vi "Find Dependency Chain.vi"() -> ()   [LabVIEW 2019, in "HawkeyeToolsMenu.lvlib"]
doc: "GUI to compare LabVIEW code between currently checked out branch with any other branch or any of its commits.\n\n(c) 2024 Soliton Technologies. All rights reserved."
uses:
  HawkeyeToolsMenu.lvlib
  cd7db559-2e0e-4359-8ea8-99399200914e.vi
  74b97984-16df-4a5a-bd9d-c6fa6725c391.vi
  vi.lib/Hawkeye/Hawkeye.lvlib
panel:
  in  "Tab Control":T1(tab)=enum."Main UI"
  out "Dependency Chain":string
  in  "Selected Dependencies":string(combo)="origin/main" caption="Dependencies"
  in  "Stop":bool
  in  "lvlib / class Path":path
  # "1. Checkout the branch of interest in your system using any method - Git command line, Desktop Git GUI Clients etc.,\n\n2. Specify the local Repository Path.\n\n3. Verify the current branch, its status and select a branch or commit based on the Compare Mode and click on Compare to display the file changes.\n\n4. Double click on a file to initiate LabVIEW code comparison.\n\n5. Once done with required comparisons, exit the tool by closing the window. The tool cleans up the temporary files added during comparison.\n\n\nNote:\n1. This tool uses LabVIEW's VI Comparison Tool which requires LabVIEW Professional Development System.\n2. It is recommended to not use other Git Clients actively when comparing files using this tool to avoid Git command related errors.\n3. It is recommended to commit all changes (working copy) before using this tool for comparison."
  # "This tool uses git diff command to identify the changes. Hence it is recommended to commit all the changes (working copy) to have them considered for comparison. For code comparison, this tool uses LabVIEW's built in VI Comparison Tool.\n\nExample: Identify changes in current branch when comparing with other branch\n\n---A---B---C---D    <== other branch\n               \\\n                 E---F      <== current branch\n\n1. We will need to identify only the file changes introduced by current branch. E and F commits are those changes in the above example (commits after the common ancestor B).\n2. For the identified file changes compare with the other branch (D) to see how it differs. These differences will be our current branch changelist.\n\nWhy only current branch changes?\nIt is most useful to see how the current branch will modify the files when it is getting merged. Best use case for displaying only current branch changelist will be for Pull Request reviews."
  # "1. VI / lvlib / class Path (Config Path)\n\n    What it is: The starting point of your dependency analysis.\n\n    How to use: Browse to or enter the absolute file path of the LabVIEW file you want to inspect.\n\n    Supported File Types: * Virtual Instruments (.vi) / LabVIEW Project Libraries (.lvlib) / LabVIEW Classes (.lvclass)\n\n2. Dependencies in Linked Project (Dropdown Menu)\n\n    What it is: A dynamically populated dropdown list showing all the valid LabVIEW files found within the scope of your linked project.\n\n    How to use: After configuring your source path, select any file from this dropdown to check if a relationship exists between it and your Config Path.\n\n3. Dependency Chain (Output Display)\n\n    What it is: The visual results area that shows the exact \"calling route\" from your Config Path to the selected dropdown dependency."
  # "Find Dependency Chain\n\nThe LabVIEW Dependency Analyzer is a specialized utility designed to map, trace, and visualize relationships between components within LabVIEW Projects, Libraries (.lvlib), and Classes (.lvclass).\n\nBy performing deep, recursive analysis on your codebase, it helps developers understand structural coupling, identify hidden linkages, and trace execution paths from a chosen source file down to its deepest sub-components.\n\nKey Features\nDeep Tracing: Automatically traverses multi-level call chains, mapping both direct and indirect dependencies."
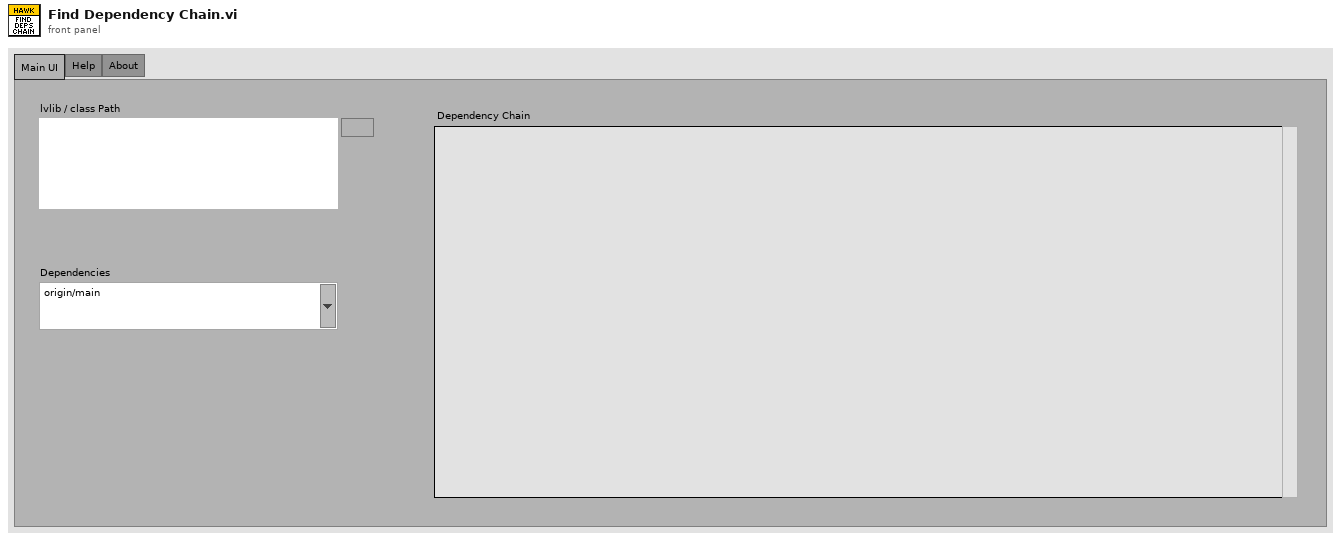
[diagram p1: front panel]
types:
  T1 = enum32{"Getting Started", "How it Works?", "Main UI", "Help", "About"}
  T2 = cluster{"lvlib / class Path":path, "Dependency Start":string, "Dependency End":string, "Repo Path":path, "All Dependency Chain":string, "Dependency Chain []":string[]}
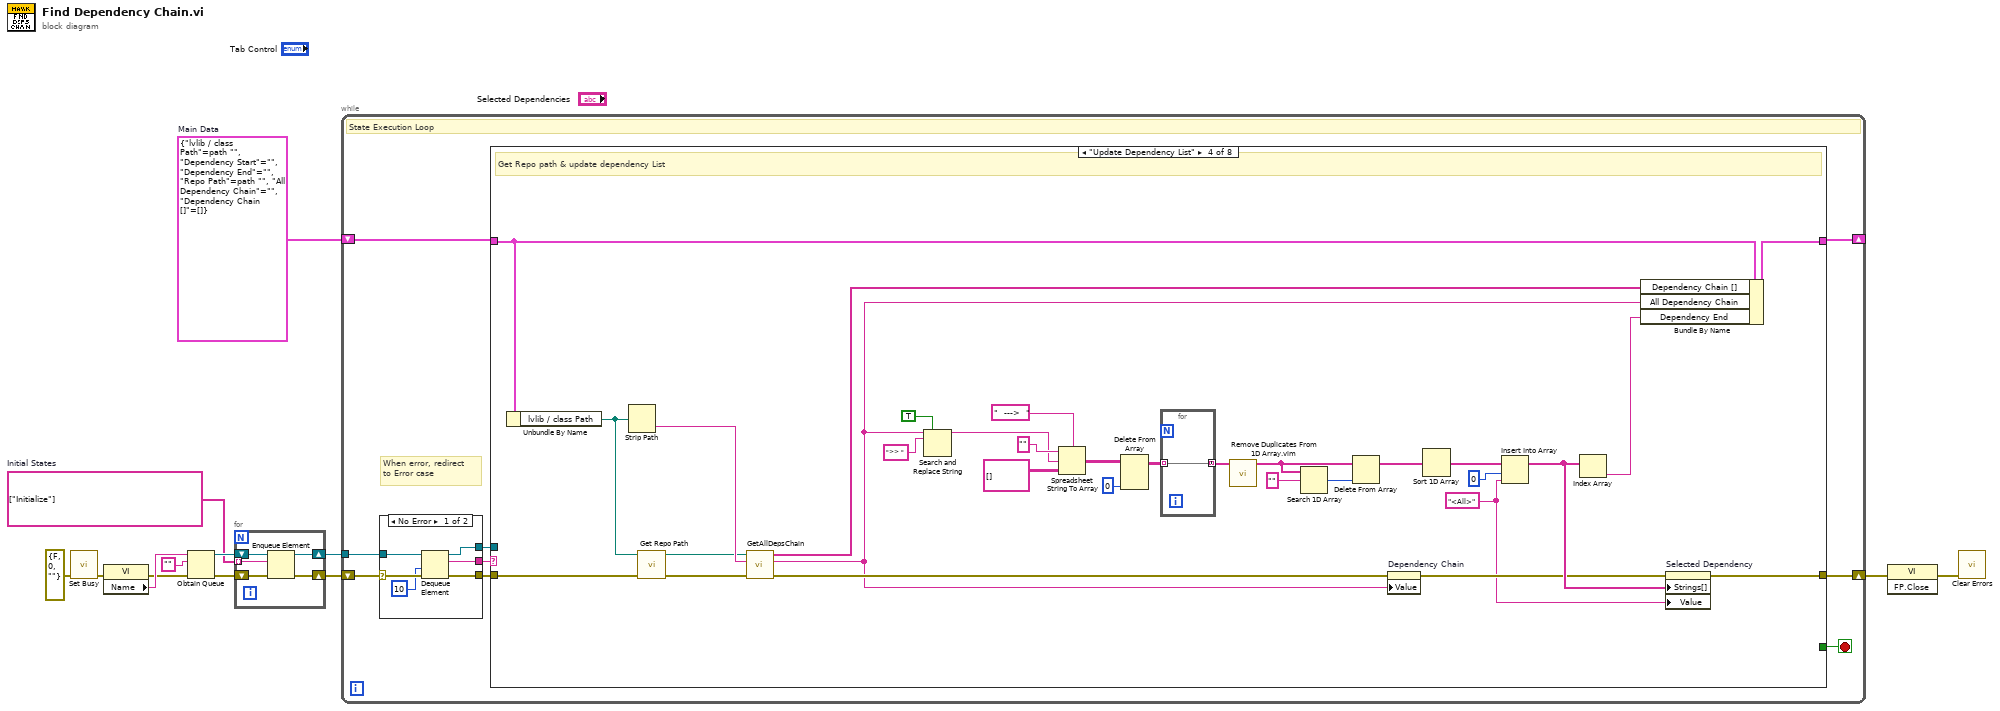
[diagram p0: block diagram]
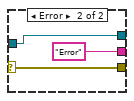
[diagram p2: hidden frame]
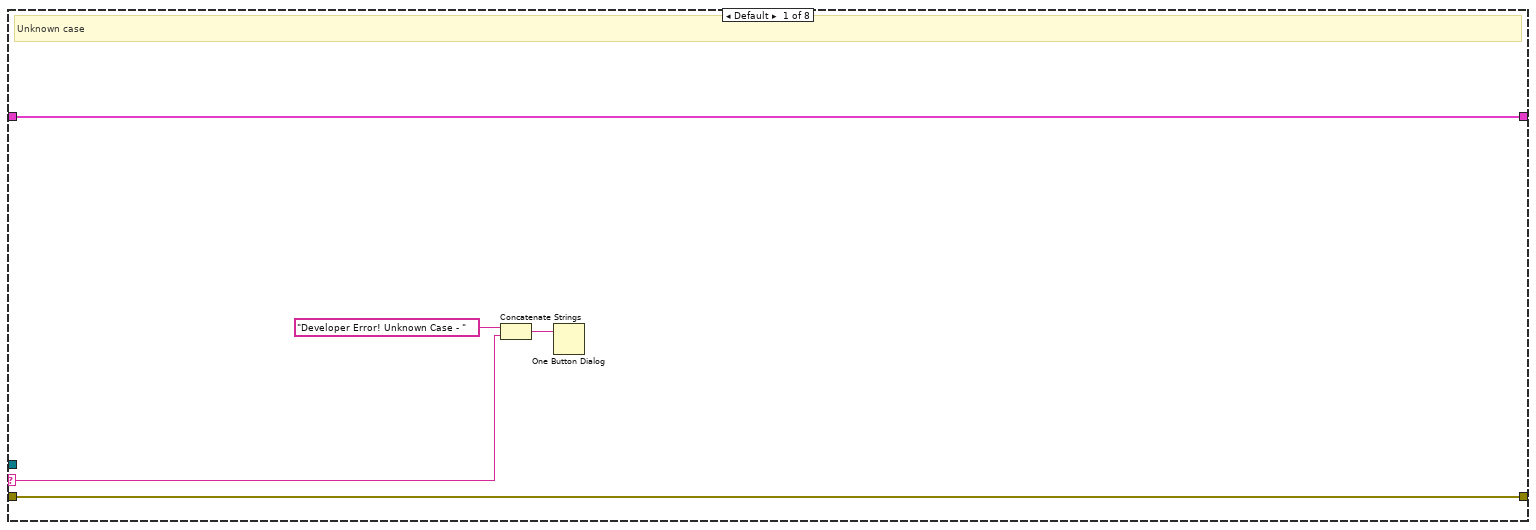
[diagram p3: hidden frame]
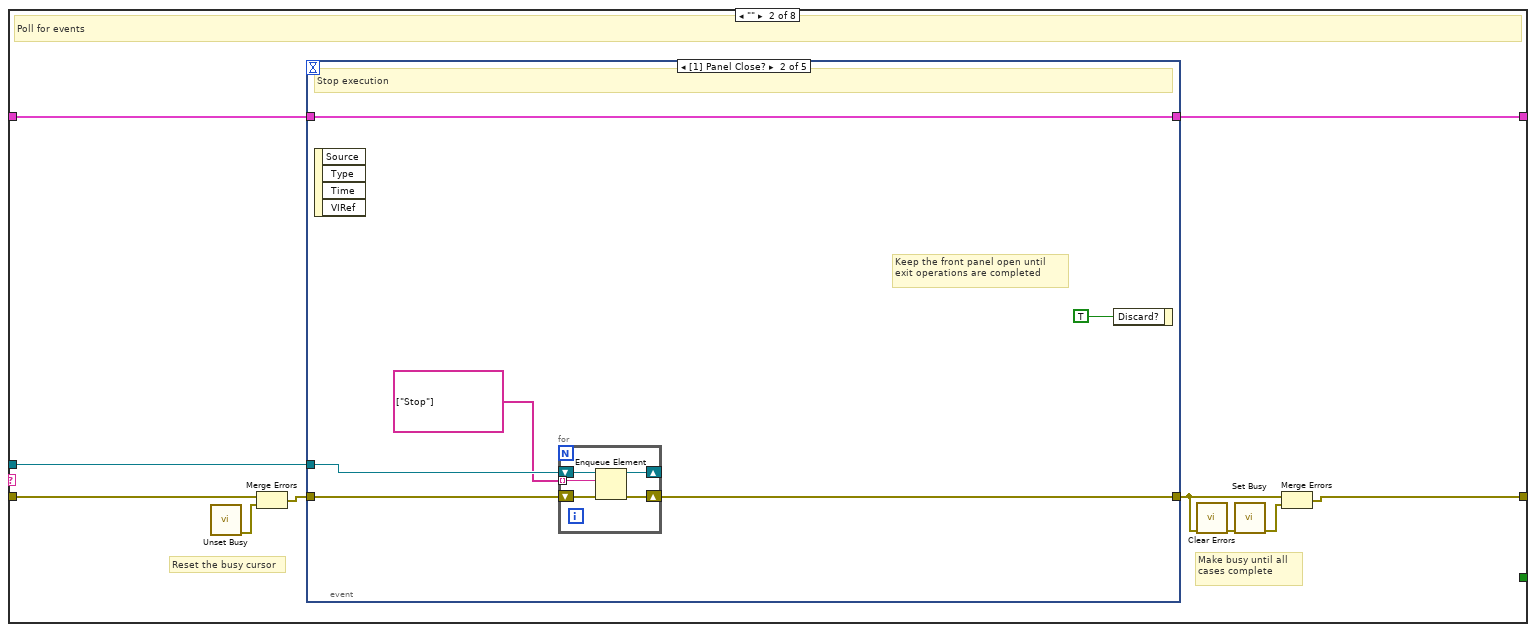
[diagram p4: hidden frame]
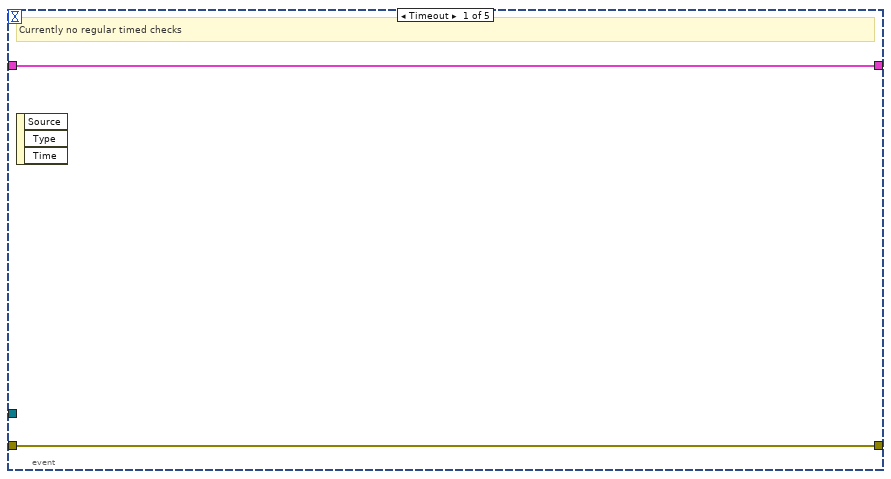
[diagram p5: hidden frame]
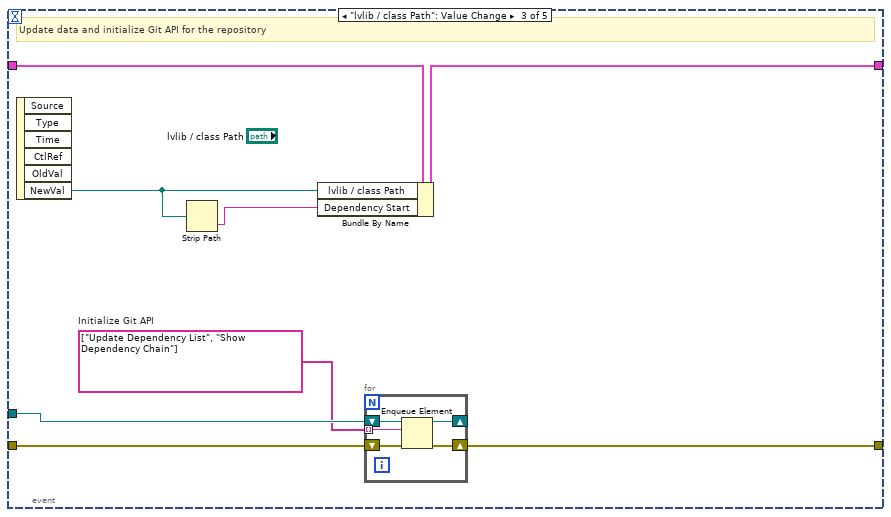
[diagram p6: hidden frame]
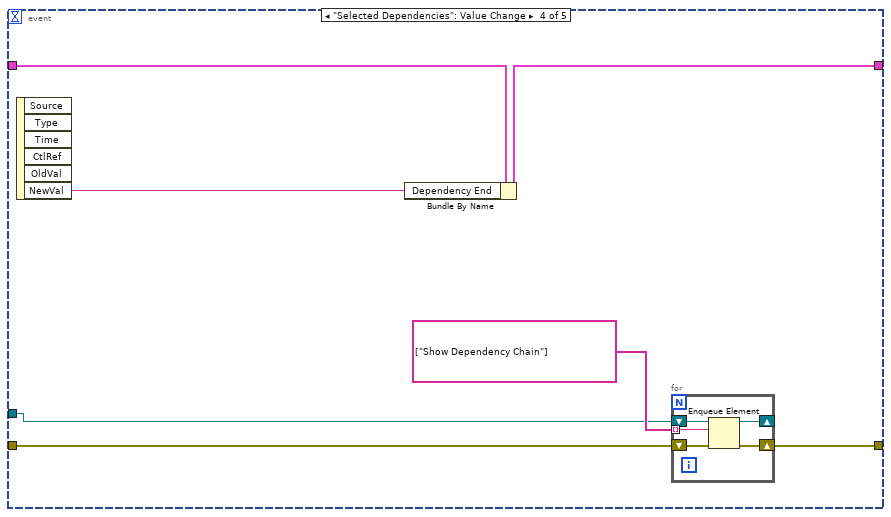
[diagram p7: hidden frame]
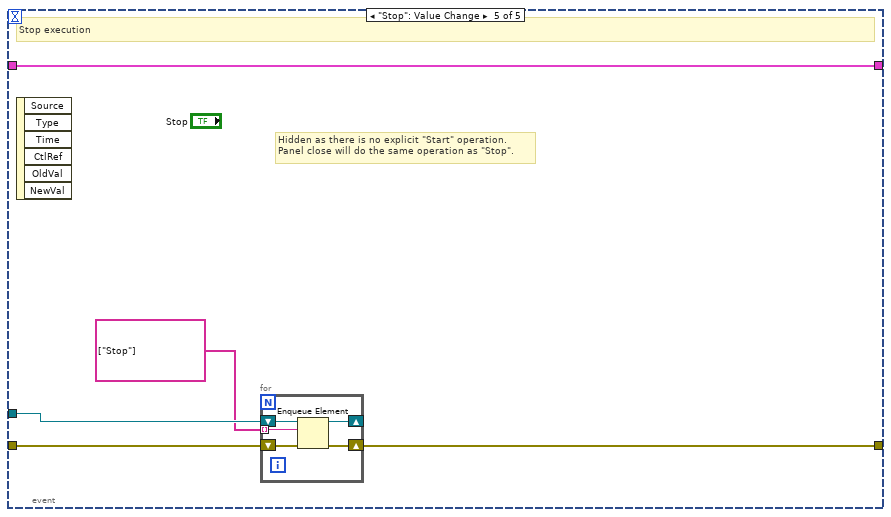
[diagram p8: hidden frame]
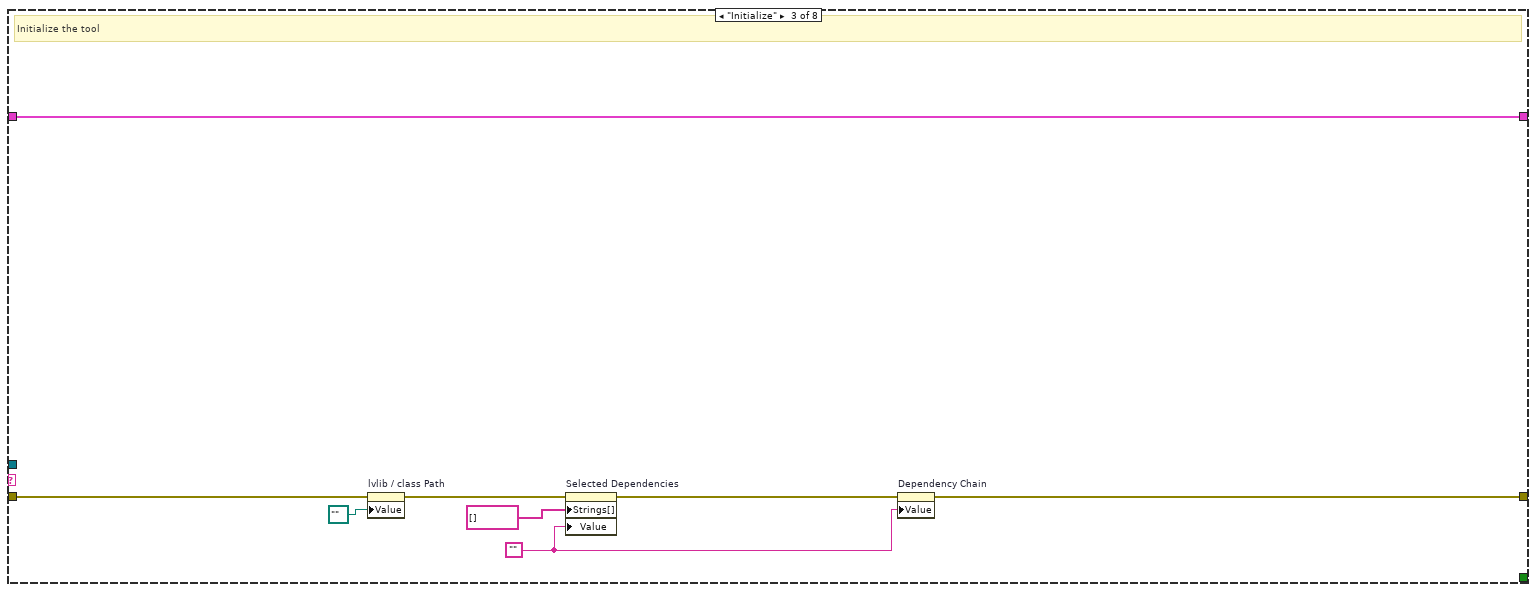
[diagram p9: hidden frame]
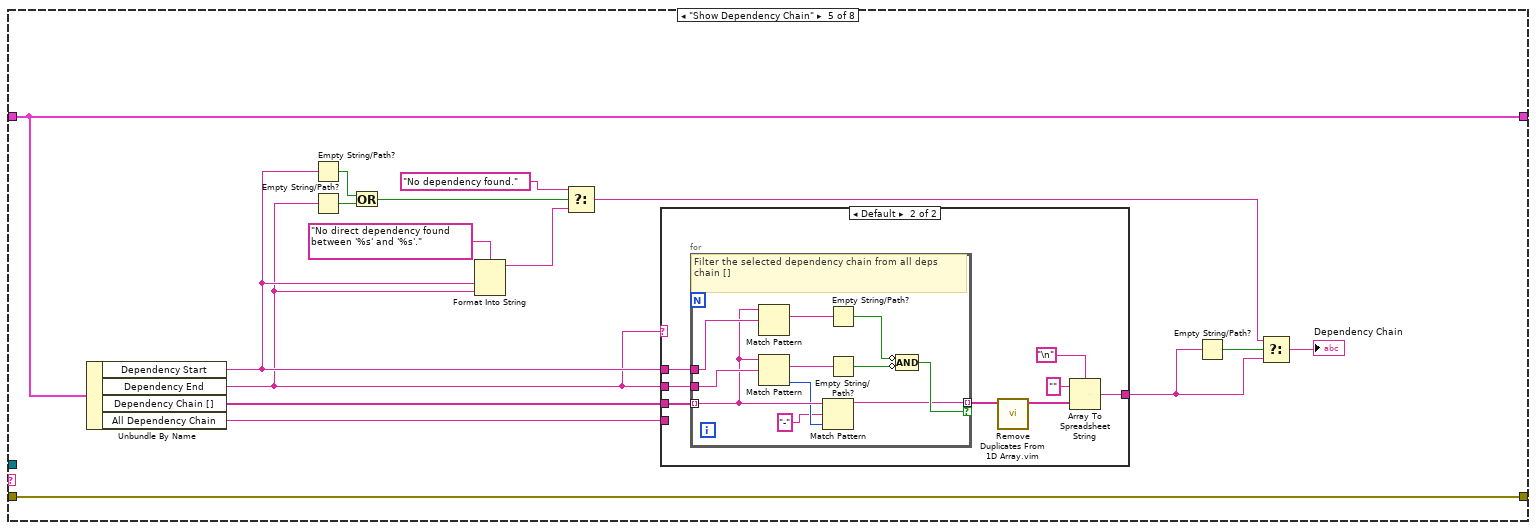
[diagram p10: hidden frame]
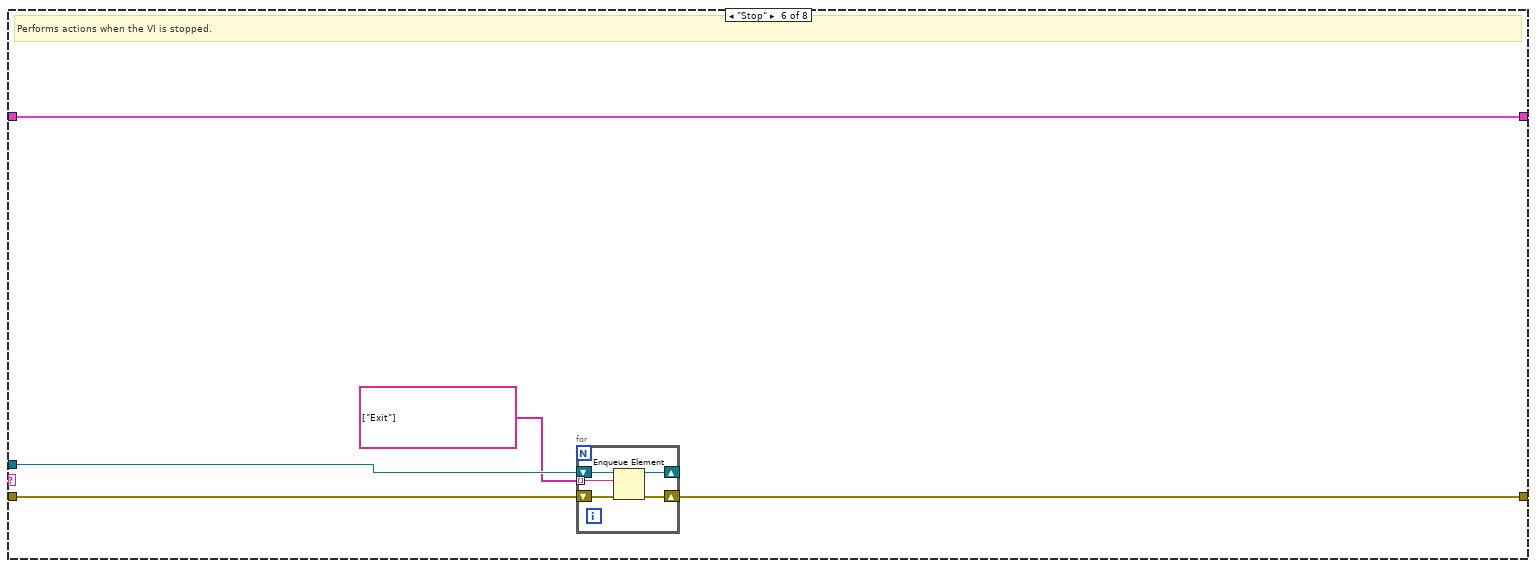
[diagram p12: hidden frame]
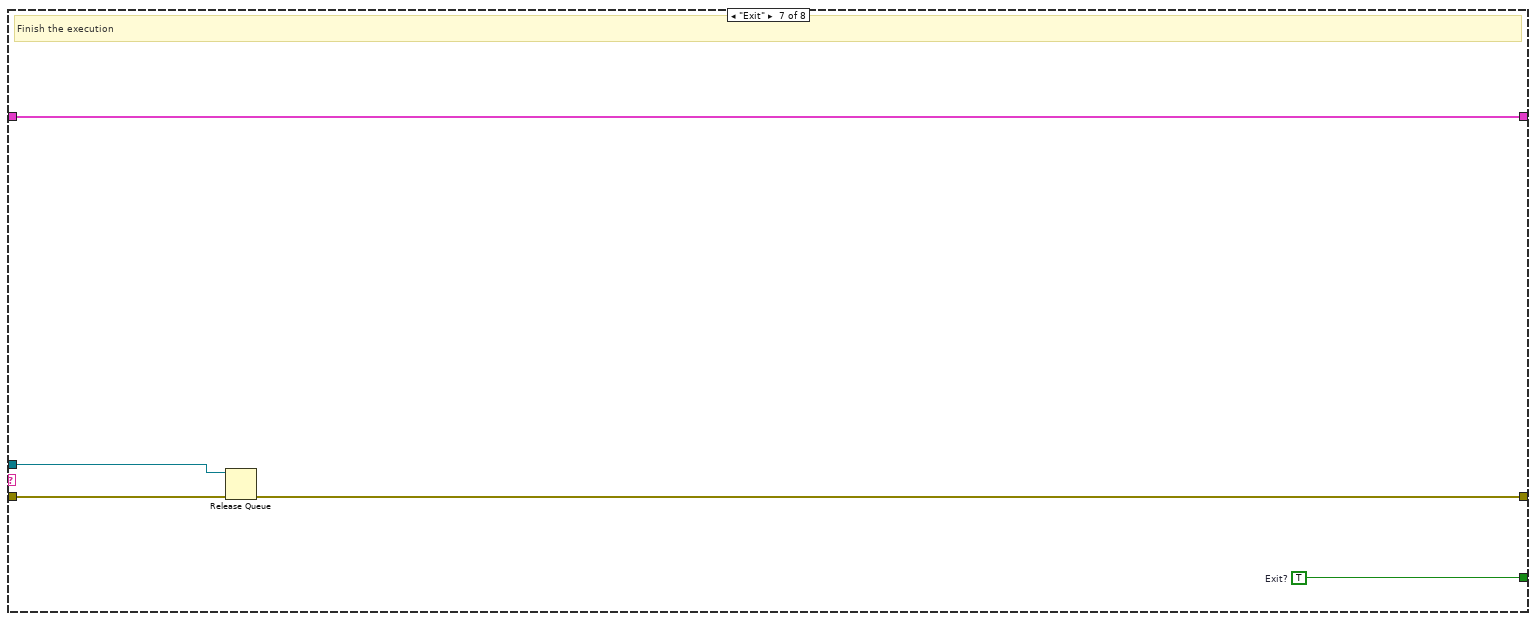
[diagram p13: hidden frame]
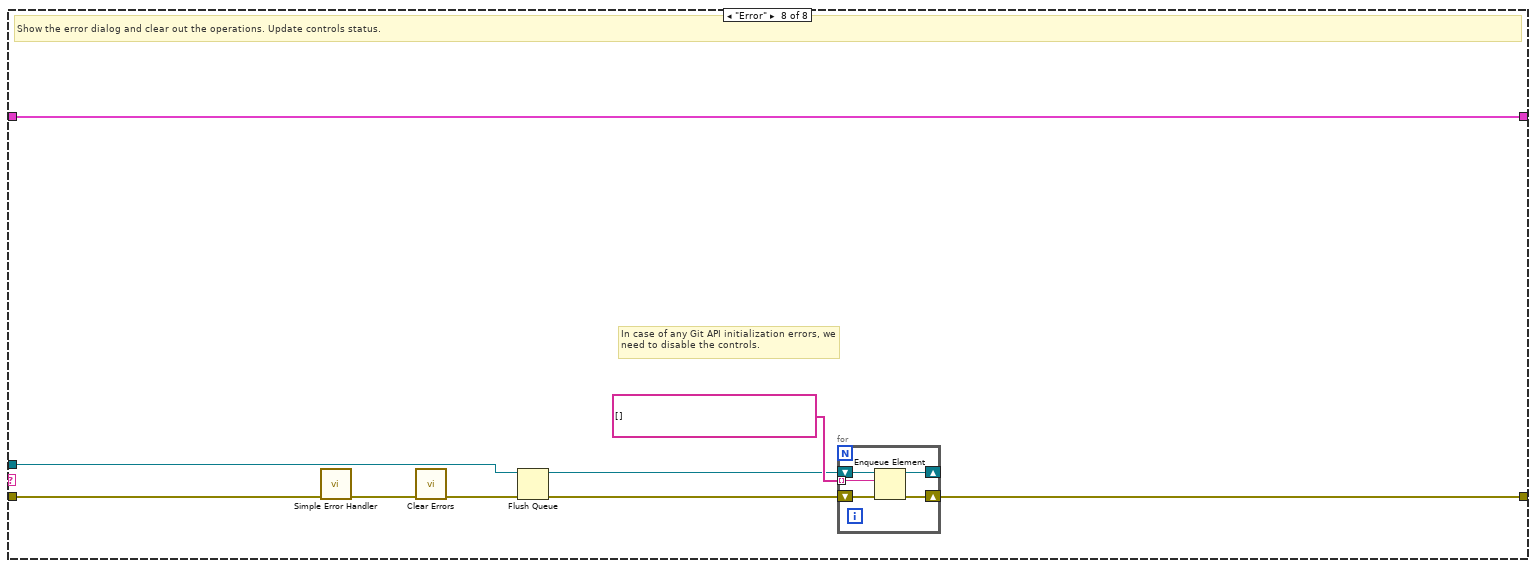
[diagram p14: hidden frame]
diagram:
  w1 = string[] ["Initialize"]  # Initial States
  w10 = T2 {"lvlib / class Path"=path "", "Dependency Start"="", "Dependency End"="", "Repo Path"=path "", "All Dependency Chain"="", "Dependency Chain []"=[]}  # Main Data
  n1 = call <vilib>:"Set Busy.vi"("error in (no error)"=errorcluster {"status"=FALSE, "code"=0, "source"=""}) -> ("error out"=w4:errorcluster)  [unwired: 9 in, 1 out]
  n2 = property class="VI"(error in=w4) -> (error out=w12:errorcluster, "Name"=w13:string)  [unwired: 1 in, 1 out]
  n3 = Obtain Queue(name (unnamed)=w13, element data type="", error in (no error)=w12) -> (queue out=w9:refnum<queue>, error out=w6:errorcluster)  [unwired: 2 in, 1 out]
  n4 = for {
    tunnel: w1 -> [w15] mode=indexing
    shift-right: [w17] -> w8
    shift-left: w6 -> [w18]
    shift-right: [w14] -> w7
    shift-left: w9 -> [w16]
    n5 = Enqueue Element(queue=w16, element=w15, error in (no error)=w18) -> (queue out=w14:refnum<queue>, error out=w17:errorcluster)  [unwired: 1 in, 1 out]
  }
  n6 = while {
    shift-right: [w19] -> w3
    shift-left: w8 -> [w21]
    tunnel: w7 -> [w22]
    shift-right: [w24] -> _
    shift-left: w10 -> [w23]
    stop <- w25 stop-if-true
    # "When error, redirect to Error case"
    # "State Execution Loop"
    n7 = case shown="No Error" w21 {
      selector: w21 -> [w30 w34]
      tunnel: [w33 "Error" ("element")] -> w27
      tunnel: [w32 w36] -> w26
      tunnel: w22 -> [w31 w36]
      tunnel: [w28 w34] -> w20
      frame No Error {
        n8 = Dequeue Element(queue=w31, timeout in ms (-1)=10, error in (no error)=w30) -> (queue out=w32:refnum<queue>, element=w33:string, error out=w28:errorcluster)  [unwired: 1 out]
      }
      frame Error {
      }
    }
    n9 = case shown="\"Update Dependency List\"" w27 {
      selector: w27 -> [w40 _ _ _ _ _ _ _]
      tunnel: w20 -> [w38 w45 w106 w121 w154 w180 w190 w198]
      tunnel: w26 -> [_ w51 _ _ _ w178 w187 w195]
      tunnel: [w38 w47 w100 w137 w154 w179 w186 w191] -> w19
      tunnel: [_ _ _ _ _ _ w188 _] -> w25
      tunnel: [w37 w49 w107 w136 w155 w177 w189 w199] -> w24
      tunnel: w23 -> [w37 w50 w107 w138 w155 w177 w189 w199]
      frame Default {
        # "Unknown case"
        n10 = Concatenate Strings("Developer Error! Unknown Case - " ("string"), w40) -> (w39:string)
        n11 = One Button Dialog(message=w39) -> ()  [unwired: 1 in, 1 out]
      }
      frame "" {
        # "Reset the busy cursor"
        # "Make busy until all cases complete"
        # "Poll for events"
        n12 = call <vilib>:"Unset Busy.vi"() -> ("error out"=w46:errorcluster)  [unwired: 11 in]
        n13 = Merge Errors(w45, w46) -> (w44:errorcluster)
        n14 = event shown="[1] Panel Close?" {
          selector: _ -> [_ _ _ _ _]
          dyn-events: _ -> [_ _ _ _ _]
          timeout: _ -> [_ _ _ _ _]
          tunnel: w44 -> [w52 w59 w70 w78 w94]
          tunnel: w51 -> [_ w58 w69 w80 w93]
          tunnel: [w52 w57 w68 w79 w92] -> w43
          tunnel: w50 -> [w53 w56 w72 w84 w91]
          tunnel: [w53 w56 w71 w83 w91] -> w49
          event Timeout {
            # "Currently no regular timed checks"
            n15 = event-data() -> ()  [unwired: 1 in, 3 out]
          }
          event Panel Close? {
            # "Keep the front panel open until exit operations are completed"
            # "Stop execution"
            n16 = event-data() -> ()  [unwired: 1 in, 4 out]
            n17 = for {
              tunnel: string[] ["Stop"] -> [w61] mode=indexing
              shift-right: [w63] -> w57
              shift-left: w59 -> [w64]
              shift-right: [w60] -> _
              shift-left: w58 -> [w62]
              n18 = Enqueue Element(queue=w62, element=w61, error in (no error)=w64) -> (queue out=w60:refnum<queue>, error out=w63:errorcluster)  [unwired: 1 in, 1 out]
            }
            n19 = event-data("Discard?"=TRUE) -> ()  [unwired: 1 in, 1 out]
          }
          event "lvlib / class Path": Value Change {
            w67 = string[] ["Update Dependency List", "Show Dependency Chain"]  # Initialize Git API
            # "Update data and initialize Git API for the repository"
            n20 = event-data() -> ("NewVal"=w66:path)  [unwired: 1 in, 5 out]
            n21 = Strip Path(path=w66) -> (name=w65:string)  [unwired: 1 out]
            n22 = Bundle By Name(cluster=w72, "lvlib / class Path"=w66, "Dependency Start"=w65) -> (w71:T2)
            n23 = for {
              tunnel: w67 -> [w74] mode=indexing
              shift-right: [w76] -> w68
              shift-left: w70 -> [w77]
              shift-right: [w73] -> _
              shift-left: w69 -> [w75]
              n24 = Enqueue Element(queue=w75, element=w74, error in (no error)=w77) -> (queue out=w73:refnum<queue>, error out=w76:errorcluster)  [unwired: 1 in, 1 out]
            }
          }
          event "Selected Dependencies": Value Change {
            n25 = event-data() -> ("NewVal"=w82:string)  [unwired: 1 in, 5 out]
            n26 = Bundle By Name(cluster=w84, "Dependency End"=w82) -> (w83:T2)
            n27 = for {
              tunnel: string[] ["Show Dependency Chain"] -> [w86] mode=indexing
              shift-right: [w88] -> w79
              shift-left: w78 -> [w89]
              shift-right: [w85] -> _
              shift-left: w80 -> [w87]
              n28 = Enqueue Element(queue=w87, element=w86, error in (no error)=w89) -> (queue out=w85:refnum<queue>, error out=w88:errorcluster)  [unwired: 1 in, 1 out]
            }
          }
          event "Stop": Value Change {
            # "Hidden as there is no explicit \"Start\" operation.\nPanel close will do the same operation as \"Stop\"."
            # "Stop execution"
            n29 = event-data() -> ()  [unwired: 1 in, 6 out]
            n30 = for {
              tunnel: string[] ["Stop"] -> [w96] mode=indexing
              shift-right: [w98] -> w92
              shift-left: w94 -> [w99]
              shift-right: [w95] -> _
              shift-left: w93 -> [w97]
              n31 = Enqueue Element(queue=w97, element=w96, error in (no error)=w99) -> (queue out=w95:refnum<queue>, error out=w98:errorcluster)  [unwired: 1 in, 1 out]
            }
          }
        }
        n32 = call <vilib>:"Clear Errors.vi"("error in (no error)"=w43) -> ("error out"=w42:errorcluster)  [unwired: 5 in, 1 out]
        n33 = call <vilib>:"Set Busy.vi"("error in (no error)"=w42) -> ("error out"=w48:errorcluster)  [unwired: 9 in, 1 out]
        n34 = Merge Errors(w43, w48) -> (w47:errorcluster)
      }
      frame "Initialize" {
        w101 = ""
        # "Initialize the tool"
        n35 = property on="lvlib / class Path" class="Path"(error in=w106, "Value"=path "" ("VI / lvlib / class Path")) -> (error out=w104:errorcluster)  [unwired: 1 in, 1 out]
        n36 = property on="Selected Dependencies" class="CmbBox"(error in=w104, "Strings[]"=string[] [] ("Strings []"), "Value"=w101) -> (error out=w102:errorcluster)  [unwired: 1 in, 1 out]
        n37 = property on="Dependency Chain" class="Str"(error in=w102, "Value"=w101) -> (error out=w100:errorcluster)  [unwired: 1 in, 1 out]
      }
      frame "Update Dependency List" {
        w108 = "<All>" ("new element/subarray")
        # "Get Repo path & update dependency List"
        n38 = Unbundle By Name(w138) -> ("lvlib / class Path"=w124:path)
        n39 = Strip Path(path=w124) -> (name=w134:string)  [unwired: 1 out]
        n40 = call "Get Repo Path.vi"("error in (no error)"=w121, "VI / lvlib / class / Folder Path"=w124) -> ("error out"=w122:errorcluster, "Repo Path"=w123:path)  [unwired: 7 in, 1 out]
        n41 = call "GetAllDepsChain.vi"("error in (no error)"=w122, "Library / Class Name"=w134, "WorkSpace / Repo path"=w123) -> ("error out"=w111:errorcluster, "All Dependency Chain"=w109:string, "Dependency Chain []"=w125:string[])  [unwired: 6 in]
        n42 = Search and Replace String(replace all?=TRUE ("replace all? (F)"), input string=w109, search string=">> ") -> (result string=w129:string)  [unwired: 5 in, 3 out]
        n43 = Spreadsheet String To Array(delimiter (Tab)="  --->  " ("search string"), format string="", spreadsheet string=w129, array type (2D Dbl)=string[][] [] ("format string")) -> (array=w126:string[][])
        n44 = Delete From Array(array=w126, index (col)=0 ("disabled index (col)")) -> (array with subset deleted=w119:string[][])  [unwired: 2 in, 1 out]
        n45 = for {
          tunnel: [w139] -> w120 mode=concatenating
          tunnel: w119 -> [w139] mode=indexing
        }
        n46 = call "Remove Duplicates From 1D Array.vim"("array"=w120) -> ("array with duplicates removed"=w116:string[])  [unwired: 10 in]
        n47 = Search 1D Array(1D array=w116, element="") -> (index of element=w117:i32)  [unwired: 1 in]
        n48 = Delete From Array(array=w116, index=w117) -> (array with subset deleted=w115:string[])  [unwired: 1 in, 1 out]
        n49 = property on="Dependency Chain" class="Str"(error in=w111, "Value"=w109) -> (error out=w110:errorcluster)  [unwired: 1 in, 1 out]
        n50 = Sort 1D Array(array=w115) -> (sorted array=w113:string[])
        n51 = Insert Into Array(array=w113, index=0, new element=w108) -> (w112:string[])
        n52 = Index Array(array=w112) -> (element=w135:string)  [unwired: 1 in]
        n53 = Bundle By Name(cluster=w138, "Dependency Chain []"=w125, "All Dependency Chain"=w109, "Dependency End"=w135) -> (w136:T2)
        n54 = property on="Selected Dependency" class="CmbBox"(error in=w110, "Strings[]"=w112, "Value"=w108) -> (error out=w137:errorcluster)  [unwired: 1 in, 1 out]
      }
      frame "Show Dependency Chain" {
        n55 = Unbundle By Name(w155) -> ("Dependency Start"=w149:string, "Dependency End"=w142:string, "Dependency Chain []"=w153:string[], "All Dependency Chain"=w140:string)
        n56 = Empty String/Path?(string/path=w149) -> (empty?=w148:bool)
        n57 = Empty String/Path?(string/path=w142) -> (empty?=w147:bool)
        n58 = Or(x=w148, y=w147) -> (x .or. y?=w146:bool)
        n59 = Format Into String(format string="No direct dependency found between '%s' and '%s'." ("t"), w149, w142) -> (resulting string=w144:string)  [unwired: 2 in, 1 out]
        n60 = Select(t="No dependency found.", s=w146, f=w144) -> (s? t:f=w143:string)
        n61 = case shown="Default" w142 {
          tunnel: w153 -> [_ w163]
          tunnel: w149 -> [_ w162]
          tunnel: w142 -> [_ w161]
          tunnel: [w156 w157] -> w141
          tunnel: w140 -> [w156 _]
          frame "<All>" {
          }
          frame Default {
            n62 = for {
              tunnel: w163 -> [w168] mode=indexing
              tunnel: w161 -> [w175]
              tunnel: w162 -> [w174]
              tunnel: [w165] -> w164 mode=indexing if=w169
              # "Filter the selected dependency chain from all deps chain []"
              n63 = Match Pattern(string=w168, regular expression=w174) -> (match substring=w173:string)  [unwired: 1 in, 3 out]
              n64 = Match Pattern(string=w168, regular expression=w175) -> (match substring=w172:string, offset past match=w167:i32)  [unwired: 1 in, 2 out]
              n65 = Match Pattern(string=w168, regular expression="-", offset (0)=w167) -> (before substring=w165:string)  [unwired: 3 out]
              n66 = Empty String/Path?(string/path=w173) -> (empty?=w171:bool)
              n67 = Empty String/Path?(string/path=w172) -> (empty?=w170:bool)
              n68 = Compound Arithmetic op=AND(invert w171, invert w170) -> (w169:bool)
            }
            n69 = call "Remove Duplicates From 1D Array.vim"("array"=w164) -> ("array with duplicates removed"=w159:string[])  [unwired: 10 in]
            n70 = Array To Spreadsheet String(delimiter (Tab)="\n", array=w159, 3:"" ("format string")) -> (spreadsheet string=w157:string)
          }
        }
        n71 = Empty String/Path?(string/path=w141) -> (empty?=w152:bool)
        n72 = Select(t=w143, s=w152, f=w141) -> (s? t:f=→"Dependency Chain":string)
      }
      frame "Stop" {
        # "Performs actions when the VI is stopped."
        n73 = for {
          tunnel: string[] ["Exit"] -> [w182] mode=indexing
          shift-right: [w184] -> w179
          shift-left: w180 -> [w185]
          shift-right: [w181] -> _
          shift-left: w178 -> [w183]
          n74 = Enqueue Element(queue=w183, element=w182, error in (no error)=w185) -> (queue out=w181:refnum<queue>, error out=w184:errorcluster)  [unwired: 1 in, 1 out]
        }
      }
      frame "Exit" {
        w188 = TRUE  # Exit?
        # "Finish the execution"
        n75 = Release Queue(queue=w187, error in (no error)=w190) -> (error out=w186:errorcluster)  [unwired: 1 in, 2 out]
      }
      frame "Error" {
        # "In case of any Git API initialization errors, we need to disable the controls."
        # "Show the error dialog and clear out the operations. Update controls status."
        n76 = call <vilib>:"Simple Error Handler.vi"("error in (no error)"=w198) -> ("error out"=w197:errorcluster)  [unwired: 4 in, 4 out]
        n77 = call <vilib>:"Clear Errors.vi"("error in (no error)"=w197) -> ("error out"=w196:errorcluster)  [unwired: 5 in, 1 out]
        n78 = Flush Queue(queue=w195, error in (no error)=w196) -> (queue out=w192:refnum<queue>, error out=w193:errorcluster)  [unwired: 1 out]
        n79 = for {
          tunnel: string[] [] -> [w201] mode=indexing
          shift-right: [w203] -> w191
          shift-left: w193 -> [w204]
          shift-right: [w200] -> _
          shift-left: w192 -> [w202]
          n80 = Enqueue Element(queue=w202, element=w201, error in (no error)=w204) -> (queue out=w200:refnum<queue>, error out=w203:errorcluster)  [unwired: 1 in, 1 out]
        }
      }
    }
  }
  n81 = invoke class="VI" method="FP.Close"(error in=w3) -> (error out=w2:errorcluster)  [unwired: 2 in, 2 out]
  n82 = call <vilib>:"Clear Errors.vi"("error in (no error)"=w2) -> ()  [unwired: 5 in, 2 out]
